vi "Initialize.vi"(8 "error in (no error)":errorcluster, 9 "Reset (True)":bool=TRUE, 10 "ID Query (True)":bool=TRUE, 11 "VISA resource name":refnum<visa-resource-name>) -> (0 "error out":errorcluster, 3 "VISA resource name out":refnum<visa-resource-name>)   [LabVIEW 2014, in "Agilent N87XX Series.lvlib"]
doc: "Establishes communication with the instrument and optionally performs an instrument identification query and/or an instrument reset. It also places the instrument in a default state needed for other instrument driver operations. Therefore, call this VI before calling other instrument driver VIs for this instrument. Generally, you need to call the Initialize VI only once at the beginning of an application."
uses:
  Agilent N87XX Series.lvlib
panel:
  # "(c) 2010 National Instruments.  ALL RIGHTS RESERVED."
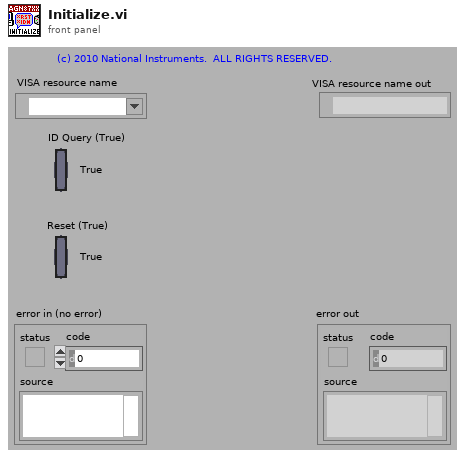
[diagram p1: front panel]
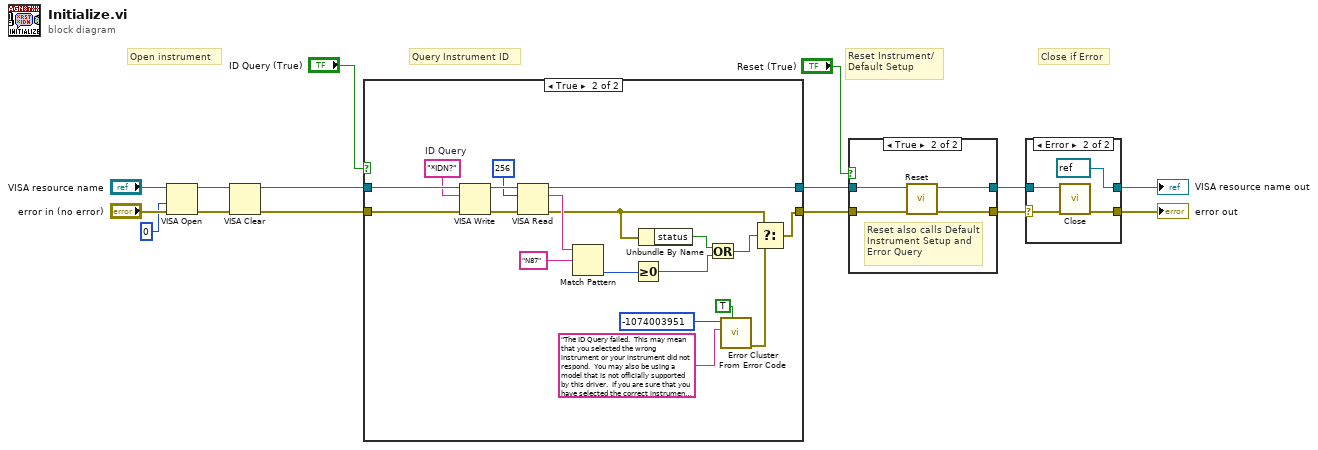
[diagram p0: block diagram]
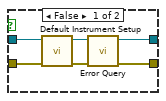
[diagram p3: hidden frame]
diagram:
  # "Close if Error"
  # "Query Instrument ID"
  # "Reset Instrument/\nDefault Setup"
  # "Open instrument"
  n1 = VISA Open(access mode=u32 0, error in (no error)="error in (no error)", VISA resource name="VISA resource name") -> (VISA resource name=w8:refnum<visa-resource-name>, error out=w7:errorcluster)  [unwired: 2 in]
  n2 = VISA Clear(VISA resource name=w8, error in (no error)=w7) -> (VISA resource name out=w2:refnum<visa-resource-name>, error out=w1:errorcluster)
  n3 = case shown="True" "ID Query (True)" {
    tunnel: [w16 w36] -> w14
    tunnel: [w17 w33] -> w15
    tunnel: w2 -> [w17 w34]
    tunnel: w1 -> [w16 w35]
    frame False {
    }
    frame True {
      w27 = "*IDN?"  # ID Query
      n4 = VISA Write(VISA resource name=w34, write buffer=w27, error in (no error)=w35) -> (VISA resource name out=w31:refnum<visa-resource-name>, error out=w30:errorcluster)  [unwired: 1 out]
      n5 = VISA Read(VISA resource name=w31, byte count=u32 256, error in (no error)=w30) -> (VISA resource name out=w33:refnum<visa-resource-name>, read buffer=w32:string, error out=w21:errorcluster)  [unwired: 1 out]
      n6 = Match Pattern(string=w32, regular expression="N87") -> (offset past match=w22:i32)  [unwired: 1 in, 3 out]
      n7 = Greater Or Equal To 0?(x=w22) -> (x >= 0?=w19:bool)
      n8 = Unbundle By Name(w21) -> ("status"=w20:bool)
      n9 = Or(x=w20, y=w19) -> (x .or. y?=w18:bool)
      n10 = call "Error Cluster From Error Code.vi"("show call chain? (False)"=TRUE, "error message (\"\")"="The ID Query failed.  This may mean that you selected the wrong instrument or your instrument did not respond.  You may also be using a model that is not officially supported by this driver.  If you are sure that you have selected the correct instrument and it is responding, try disabling the ID Query." ("Source (VI Name)"), "error code (0)"=-1074003951 ("Code")) -> ("error out"=w26:errorcluster)  [unwired: 6 in]
      n11 = Select(t=w21, s=w18, f=w26) -> (s? t:f=w36:errorcluster)
    }
  }
  n12 = case shown="True" "Reset (True)" {
    tunnel: w14 -> [w41 w43]
    tunnel: [w38 w46] -> w3
    tunnel: w15 -> [w42 w44]
    tunnel: [w39 w45] -> w4
    frame False {
      n13 = call "Default Instrument Setup.vi"("error in (no error)"=w41, "VISA resource name"=w42) -> ("error out"=w37:errorcluster, "VISA resource name out"=w40:refnum<visa-resource-name>)  [unwired: 8 in]
      n14 = call "Error Query.vi"("error in (no error)"=w37, "VISA resource name"=w40) -> ("error out"=w38:errorcluster, "VISA resource name out"=w39:refnum<visa-resource-name>)  [unwired: 6 in, 2 out]
    }
    frame True {
      # "Reset also calls Default Instrument Setup and Error Query"
      n15 = call "Reset.vi"("error in (no error)"=w43, "VISA resource name"=w44) -> ("error out"=w46:errorcluster, "VISA resource name out"=w45:refnum<visa-resource-name>)  [unwired: 8 in]
    }
  }
  n16 = case shown="Error" w3 {
    selector: w3 -> [w47 w50]
    tunnel: w4 -> [w48 w51]
    tunnel: [w48 refnum<visa-resource-name> refnum ("VISA resource name out")] -> w6
    tunnel: [w47 w52] -> w5
    frame No Error {
    }
    frame Error {
      n17 = call "Close.vi"("error in (no error)"=w50, "VISA resource name"=w51) -> ("error out"=w52:errorcluster)  [unwired: 9 in]
    }
  }
  "VISA resource name out" <- w6
  "error out" <- w5
